vi "Set Loop Period.vi"() -> ()   [LabVIEW 2019]
panel:
  in  "stop":bool
  out "Waveform Chart":dbl(graph)=-0.15643446504023392
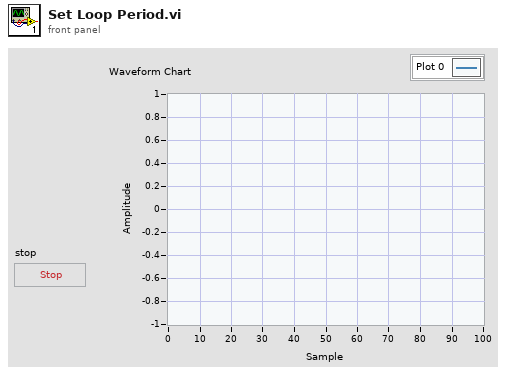
[diagram p1: front panel]
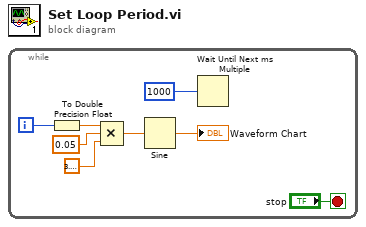
[diagram p0: block diagram]
diagram:
  n1 = while {
    i -> [w8]
    stop <- "stop" stop-if-true
    n2 = To Double Precision Float(number=w8) -> (double precision float=w7:dbl)
    n3 = Compound Arithmetic op=MULTIPLY(w7, 0.05, 3.141592653589793) -> (w4:dbl)
    n4 = Sine(x=w4) -> (sin(x)=→"Waveform Chart":dbl)
    n5 = Wait Until Next ms Multiple(millisecond multiple=u32 1000) -> ()  [unwired: 1 out]
  }
